vi "Update Test Limits.vi"(7 "Die_Variant":i32=29, 10 "TestNumbers_to_Udate_Limits":dbl[](array[numeric])=[100.0], 11 "Master_Limits_Info":string[][](array[string])=[["Test Number", "Generic Test Name\n", "Variant", "HV_Trim_Settings\n", "Low Limit\n", "High Limit\n"], ["100", "test1", "26", "10,11,12,13", "10", "20"], ["103", "est2", "29", "31,30,0,21", "30", "40"]]) -> (2 "Updated_USL":dbl[](array[numeric])=[100.0], 3 "Updated_LSL":dbl[](array[numeric])=[100.0])   [LabVIEW 2013]
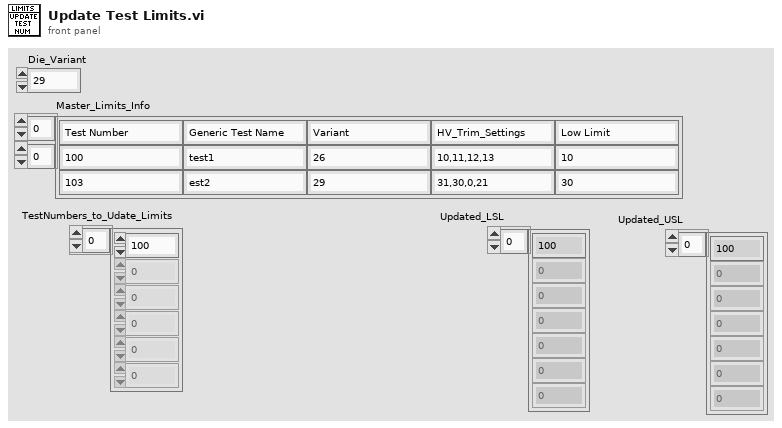
[diagram p1: front panel]
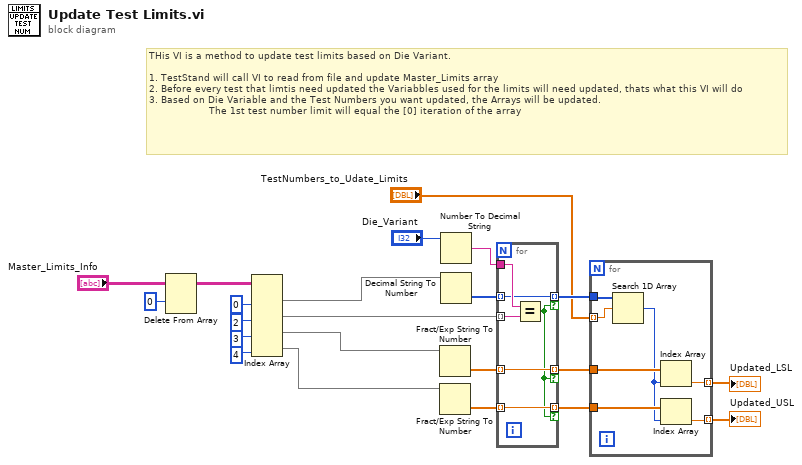
[diagram p0: block diagram]
diagram:
  # "THis VI is a method to update test limits based on Die Variant.\n\n1. TestStand will call VI to read from file and update Master_Limits array\n2. Before every test that limtis need updated the Variabbles used for the limits will need updated, thats what this VI will do\n3. Based on Die Variable and the Test Numbers you want updated, the Arrays will be updated.\n                    The 1st test number limit will equal the [0] iteration of the array"
  n1 = Delete From Array(array="Master_Limits_Info", index (row)=0) -> (array with subset deleted=w20:string[][])  [unwired: 2 in, 1 out]
  n2 = Index Array(array=w20, index (col) #1=0 ("disabled index (col)"), index (col) #2=2 ("index (col)"), index (col) #3=3 ("index (col)"), index (col) #4=4 ("index (col)")) -> (element #1=w16:string[], element #2=w14:string[], element #3=w13:string[], element #4=w12:string[])  [unwired: 4 in]
  n3 = Fract/Exp String To Number(string=w13) -> (number=w18:dbl[])  [unwired: 3 in, 1 out]
  n4 = Fract/Exp String To Number(string=w12) -> (number=w17:dbl[])  [unwired: 3 in, 1 out]
  n5 = Number To Decimal String(number="Die_Variant") -> (decimal integer string=w7:string)  [unwired: 1 in]
  n6 = Decimal String To Number(string=w16) -> (number=w15:i32[])  [unwired: 2 in, 1 out]
  n7 = for {
    tunnel: w14 -> [w26] mode=indexing
    tunnel: w7 -> [w25]
    tunnel: w18 -> [w28] mode=indexing
    tunnel: w17 -> [w27] mode=indexing
    tunnel: [w28] -> w5 mode=indexing if=w23
    tunnel: [w27] -> w4 mode=indexing if=w23
    tunnel: w15 -> [w24] mode=indexing
    tunnel: [w24] -> w6 mode=indexing if=w23
    n8 = Equal?(x=w25, y=w26) -> (x = y?=w23:bool)
  }
  n9 = for {
    tunnel: w6 -> [w35]
    tunnel: w5 -> [w33]
    tunnel: w4 -> [w32]
    tunnel: "TestNumbers_to_Udate_Limits" -> [w34] mode=indexing
    tunnel: [w30] -> w2 mode=indexing
    tunnel: [w29] -> w1 mode=indexing
    n10 = Search 1D Array(1D array=w35, element=w34) -> (index of element=w31:i32)  [unwired: 1 in]
    n11 = Index Array(array=w33, index=w31) -> (element=w30:dbl)
    n12 = Index Array(array=w32, index=w31) -> (element=w29:dbl)
  }
  "Updated_LSL" <- w2
  "Updated_USL" <- w1
